vi "CtrlTreeRestoreState.vi"(8 "error in (no error)":errorcluster, 10 "State":T1={"Closed Nodes"=[], "Selection"=[], "Defer Panel Update"=TRUE}, 11 "TreeControl in":refnum<vi>) -> (0 "error out":errorcluster, 3 "TreeControl out":refnum<vi>)   [LabVIEW 2020]
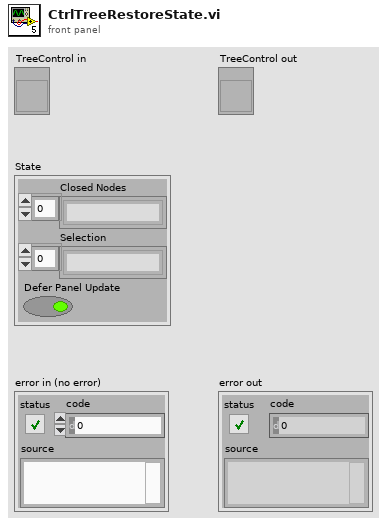
[diagram p1: front panel]
types:
  T1 = cluster{"Closed Nodes":string[], "Selection":string[], "Defer Panel Update":bool}
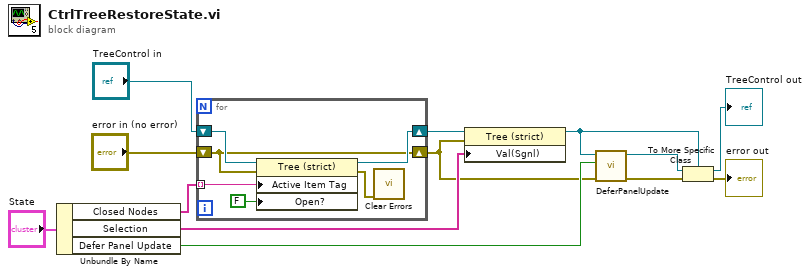
[diagram p0: block diagram]
diagram:
  n1 = Unbundle By Name("State") -> ("Closed Nodes"=w10:string[], "Selection"=w9:string[], "Defer Panel Update"=w3:bool)
  n2 = for {
    tunnel: w10 -> [w18] mode=indexing
    shift-right: [w16] -> w13
    shift-left: "TreeControl in" -> [w17]
    shift-right: [w15] -> w2
    shift-left: "error in (no error)" -> [w15]
    n3 = property class="Tree (strict)"(reference=w17, error in=w15, "Active Item Tag"=w18, "Open?"=FALSE ("Active Item:Open?")) -> (reference out=w16:refnum<vi>, error out=w14:errorcluster)
    n4 = call <vilib>:"Clear Errors.vi"("error in (no error)"=w14) -> ()  [unwired: 5 in, 2 out]
  }
  n5 = property class="Tree (strict)"(reference=w13, error in=w2, "Val(Sgnl)"=w9) -> (reference out=w6:refnum<vi>)  [unwired: 1 out]
  n6 = call "DeferPanelUpdate.vi"("error in (no error)"=w2, "Defer Panel Updates (T)"=w3, "Control in"=w6) -> ("error out"=w7:errorcluster, "Control out"=w4:refnum<vi>)  [unwired: 6 in, 1 out]
  n7 = To More Specific Class(target class=w6, reference=w4, error in=w7) -> (specific class reference=→"TreeControl out":refnum<vi>, error out=→"error out":errorcluster)
